vi "Shooter Oper.vi"   [LabVIEW 2016]
uses:
  Robot Global Data.vi
types:
  T1 = typedef "WPI_DriverStationRobotMode2.ctl" = enum16{"Autonomous Disabled", "Autonomous Enabled", "Teleop Disabled", "Teleop Enabled", "Disconnected", "Finish", "Test Disabled", "Test Enabled", "Emergency Stopped"}
  T2 = typedef "WPI_MotorControlDeviceRef.ctl" = cluster{"DeviceStatus":errorcluster, "Type":T3, "PWM":cluster{"PWM Channel":T4, "DeadBand":T5}, "CAN":cluster{"Device Number":u8, "SetOutput VI Ref":variant, "GetOutput VI Ref":variant, "Enable VI Ref":variant, "Disable VI Ref":variant, "Data":variant}, "Invert":bool}
  T3 = typedef "WPI_MotorControlType.ctl" = enum16{"PWM", "CAN"}
  T4 = typedef "FPGA_DIOPWMChannel.ctl" = enum8{"PWM 0", "PWM 1", "PWM 2", "PWM 3", "PWM 4", "PWM 5", "PWM 6", "PWM 7", "PWM 8", "PWM 9", "PWM MXP 0", "PWM MXP 1", "PWM MXP 2", "PWM MXP 3", "PWM MXP 4", "PWM MXP 5", "PWM MXP 6", "PWM MXP 7", "PWM MXP 8", "PWM MXP 9", "Invalid"}
  T5 = typedef "WPI_PWMDeadband.ctl" = cluster{"Name":string, "maxPositivePwm":i32, "minPositivePwm":i32, "centerPwm":i32, "maxNegativePwm":i32, "minNegativePwm":i32, "angularRange":u16}
  T6 = enum16{"Shooter 1 Speed Increase", "Shooter 1 Speed Decrease", "Shooter 2 Speed Increase", "Shooter 2 Speed Decrease", "Nothing Changed", "Set Zero"}
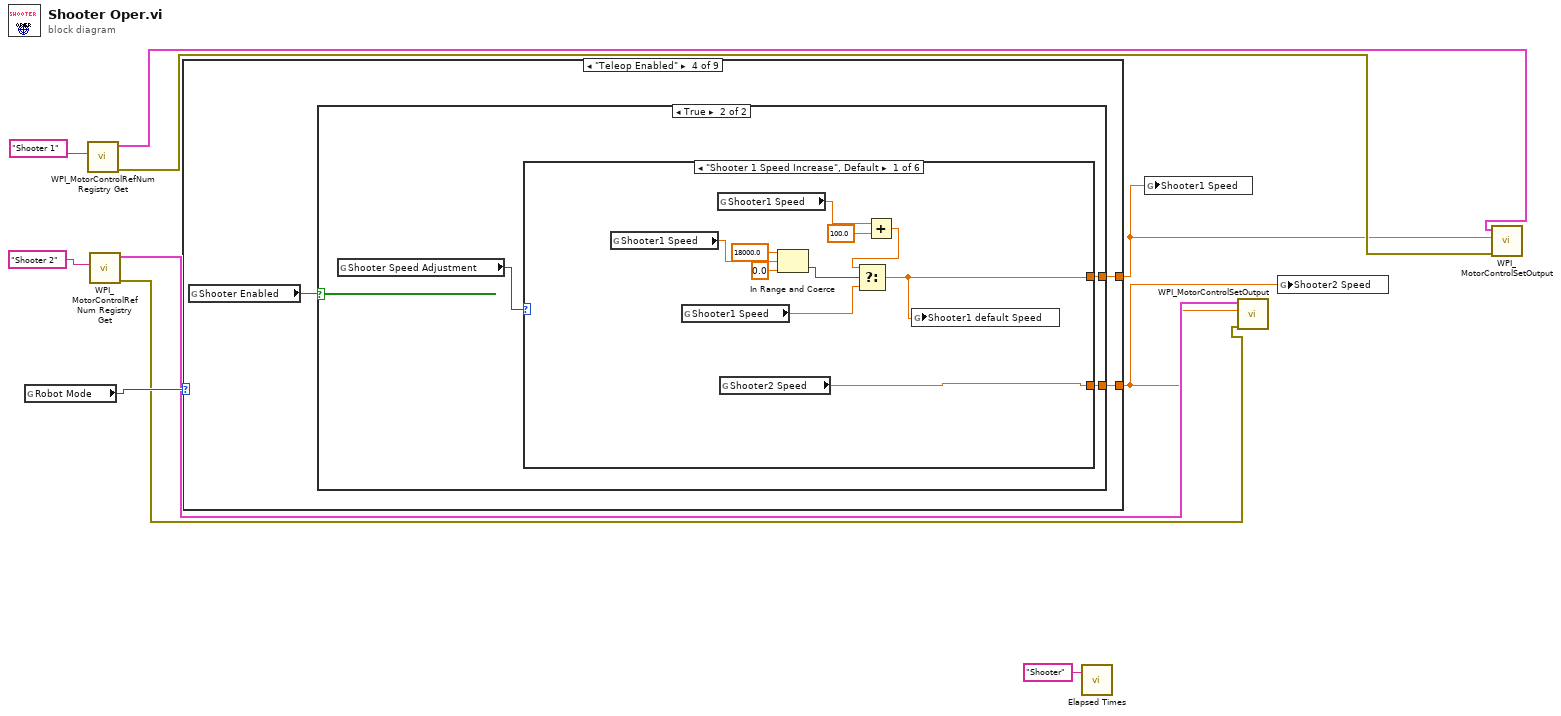
[diagram p0: block diagram]
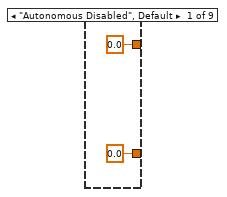
[diagram p2: hidden frame]
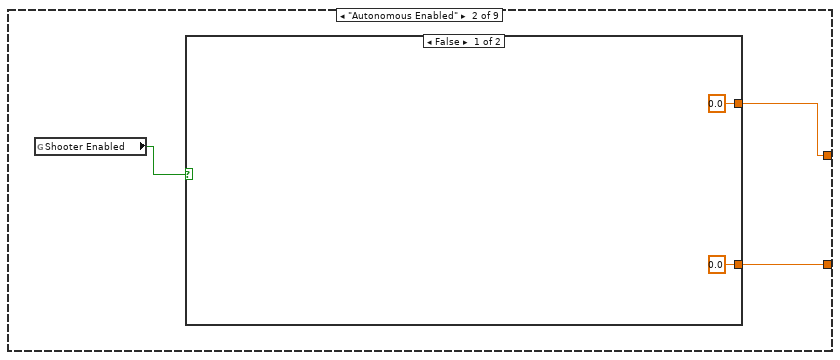
[diagram p3: hidden frame]
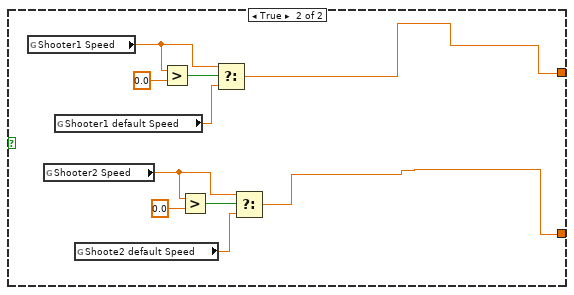
[diagram p4: hidden frame]
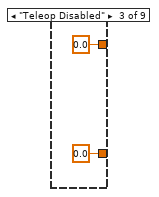
[diagram p5: hidden frame]
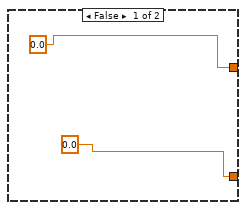
[diagram p6: hidden frame]
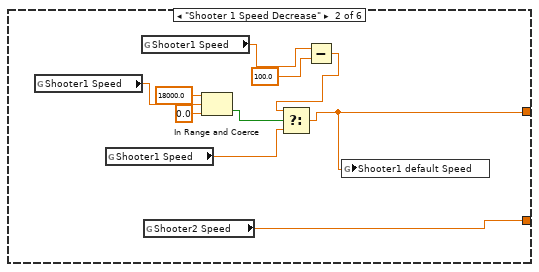
[diagram p7: hidden frame]
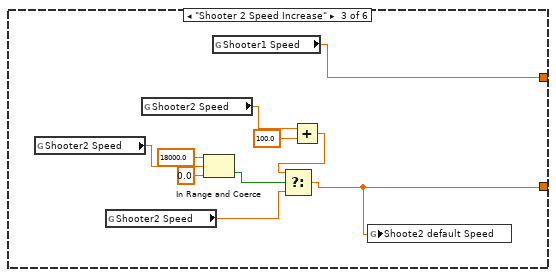
[diagram p8: hidden frame]
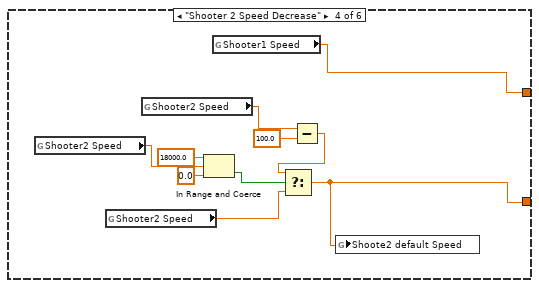
[diagram p9: hidden frame]
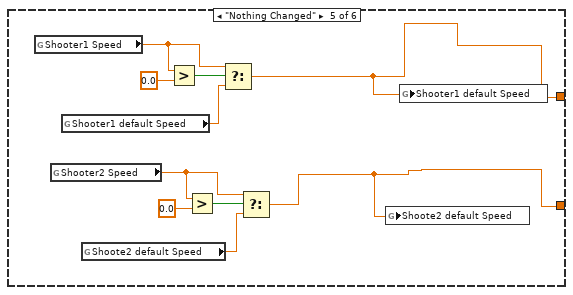
[diagram p10: hidden frame]
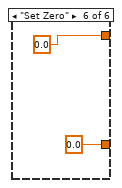
[diagram p11: hidden frame]
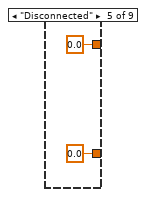
[diagram p12: hidden frame]
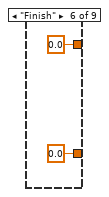
[diagram p13: hidden frame]
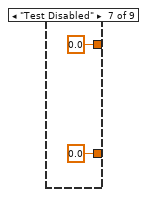
[diagram p14: hidden frame]
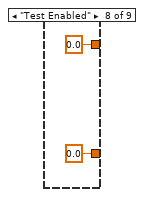
[diagram p15: hidden frame]
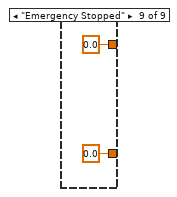
[diagram p16: hidden frame]
diagram:
  n1 = global read "Robot Global Data.vi" "Robot Mode"() -> (w8:T1)
  n2 = call <vilib>:"WPI_MotorControlRefNum Registry Get.vi"("refnum name"="Shooter 1") -> ("error out"=w5:errorcluster, "MotorControlDevRef"=w7:T2)  [unwired: 9 in]
  n3 = call <vilib>:"WPI_MotorControlRefNum Registry Get.vi"("refnum name"="Shooter 2") -> ("error out"=w4:errorcluster, "MotorControlDevRef"=w6:T2)  [unwired: 9 in]
  n4 = case shown="\"Teleop Enabled\"" w8 {
    tunnel: [0.0 ("Shooter1 Speed") w13 0.0 ("Shooter1 Speed") w31 0.0 ("Shooter1 Speed") 0.0 ("Shooter1 Speed") 0.0 ("Shooter1 Speed") 0.0 ("Shooter1 Speed") 0.0 ("Shooter1 Speed")] -> w3
    tunnel: [0.0 ("Shooter2 Speed") w14 0.0 ("Shooter2 Speed") w30 0.0 ("Shooter2 Speed") 0.0 ("Shooter2 Speed") 0.0 ("Shooter2 Speed") 0.0 ("Shooter2 Speed") 0.0 ("Shooter2 Speed")] -> w2
    frame "Autonomous Disabled", Default {
    }
    frame "Autonomous Enabled" {
      n5 = global read "Robot Global Data.vi" "Shooter Enabled"() -> (w15:bool)
      n6 = case shown="False" w15 {
        tunnel: [0.0 ("Shooter2 Speed") w19] -> w14
        tunnel: [0.0 ("Shooter1 Speed") w18] -> w13
        frame False {
        }
        frame True {
          n7 = global read "Robot Global Data.vi" "Shooter1 Speed"() -> (w25:dbl)
          n8 = global read "Robot Global Data.vi" "Shooter2 Speed"() -> (w21:dbl)
          n9 = global read "Robot Global Data.vi" "Shooter1 default Speed"() -> (w24:dbl)
          n10 = global read "Robot Global Data.vi" "Shoote2 default Speed"() -> (w20:dbl)
          n11 = Greater?(x=w25, y=0.0) -> (0:w26:bool)
          n12 = Greater?(x=w21, y=0.0) -> (0:w22:bool)
          n13 = Select(t=w25, s=w26, f=w24) -> (s? t:f=w18:dbl)
          n14 = Select(t=w21, s=w22, f=w20) -> (s? t:f=w19:dbl)
        }
      }
    }
    frame "Teleop Disabled" {
    }
    frame "Teleop Enabled" {
      n15 = global read "Robot Global Data.vi" "Shooter Enabled"() -> (w32:bool)
      n16 = case shown="True" w32 {
        tunnel: [0.0 ("Shooter1 Speed") w36] -> w31
        tunnel: [0.0 ("Shooter2 Speed") w35] -> w30
        frame False {
        }
        frame True {
          n17 = global read "Robot Global Data.vi" "Shooter Speed Adjustment"() -> (w37:T6)
          n18 = case shown="\"Shooter 1 Speed Increase\", Default" w37 {
            tunnel: [w38 w48 w59 w69 w79 0.0 ("Shooter1 Speed")] -> w36
            tunnel: [w39 w49 w58 w68 w78 0.0 ("Shooter2 Speed")] -> w35
            frame "Shooter 1 Speed Increase", Default {
              n19 = global read "Robot Global Data.vi" "Shooter1 Speed"() -> (w47:dbl)
              n20 = global read "Robot Global Data.vi" "Shooter1 Speed"() -> (w43:dbl)
              n21 = global read "Robot Global Data.vi" "Shooter1 Speed"() -> (w42:dbl)
              n22 = global read "Robot Global Data.vi" "Shooter2 Speed"() -> (w39:dbl)
              n23 = In Range and Coerce(upper limit=18000.0, x=w47, lower limit=0.0) -> (In Range?=w44:bool)  [unwired: 1 out]
              n24 = Add(x=w42, y=100.0) -> (x+y=w40:dbl)
              n25 = Select(t=w40, s=w44, f=w43) -> (s? t:f=w38:dbl)
              n26 = global write "Robot Global Data.vi" "Shooter1 default Speed"(w38) -> ()
            }
            frame "Shooter 1 Speed Decrease" {
              n27 = global read "Robot Global Data.vi" "Shooter1 Speed"() -> (w57:dbl)
              n28 = global read "Robot Global Data.vi" "Shooter1 Speed"() -> (w53:dbl)
              n29 = global read "Robot Global Data.vi" "Shooter1 Speed"() -> (w52:dbl)
              n30 = global read "Robot Global Data.vi" "Shooter2 Speed"() -> (w49:dbl)
              n31 = In Range and Coerce(upper limit=18000.0, x=w57, lower limit=0.0) -> (In Range?=w54:bool)  [unwired: 1 out]
              n32 = Subtract(x=w52, y=100.0) -> (x-y=w50:dbl)
              n33 = Select(t=w50, s=w54, f=w53) -> (s? t:f=w48:dbl)
              n34 = global write "Robot Global Data.vi" "Shooter1 default Speed"(w48) -> ()
            }
            frame "Shooter 2 Speed Increase" {
              n35 = global read "Robot Global Data.vi" "Shooter2 Speed"() -> (w67:dbl)
              n36 = global read "Robot Global Data.vi" "Shooter2 Speed"() -> (w63:dbl)
              n37 = global read "Robot Global Data.vi" "Shooter2 Speed"() -> (w62:dbl)
              n38 = In Range and Coerce(upper limit=18000.0, x=w67, lower limit=0.0) -> (In Range?=w64:bool)  [unwired: 1 out]
              n39 = global read "Robot Global Data.vi" "Shooter1 Speed"() -> (w59:dbl)
              n40 = Add(x=w62, y=100.0) -> (x+y=w60:dbl)
              n41 = Select(t=w60, s=w64, f=w63) -> (s? t:f=w58:dbl)
              n42 = global write "Robot Global Data.vi" "Shoote2 default Speed"(w58) -> ()
            }
            frame "Shooter 2 Speed Decrease" {
              n43 = global read "Robot Global Data.vi" "Shooter2 Speed"() -> (w77:dbl)
              n44 = global read "Robot Global Data.vi" "Shooter2 Speed"() -> (w73:dbl)
              n45 = global read "Robot Global Data.vi" "Shooter2 Speed"() -> (w72:dbl)
              n46 = In Range and Coerce(upper limit=18000.0, x=w77, lower limit=0.0) -> (In Range?=w74:bool)  [unwired: 1 out]
              n47 = global read "Robot Global Data.vi" "Shooter1 Speed"() -> (w69:dbl)
              n48 = Subtract(x=w72, y=100.0) -> (x-y=w70:dbl)
              n49 = Select(t=w70, s=w74, f=w73) -> (s? t:f=w68:dbl)
              n50 = global write "Robot Global Data.vi" "Shoote2 default Speed"(w68) -> ()
            }
            frame "Nothing Changed" {
              n51 = global read "Robot Global Data.vi" "Shooter1 Speed"() -> (w85:dbl)
              n52 = global read "Robot Global Data.vi" "Shooter2 Speed"() -> (w81:dbl)
              n53 = global read "Robot Global Data.vi" "Shooter1 default Speed"() -> (w84:dbl)
              n54 = global read "Robot Global Data.vi" "Shoote2 default Speed"() -> (w80:dbl)
              n55 = Greater?(x=w85, y=0.0) -> (0:w86:bool)
              n56 = Greater?(x=w81, y=0.0) -> (0:w82:bool)
              n57 = Select(t=w85, s=w86, f=w84) -> (s? t:f=w79:dbl)
              n58 = Select(t=w81, s=w82, f=w80) -> (s? t:f=w78:dbl)
              n59 = global write "Robot Global Data.vi" "Shoote2 default Speed"(w78) -> ()
              n60 = global write "Robot Global Data.vi" "Shooter1 default Speed"(w79) -> ()
            }
            frame "Set Zero" {
            }
          }
        }
      }
    }
    frame "Disconnected" {
    }
    frame "Finish" {
    }
    frame "Test Disabled" {
    }
    frame "Test Enabled" {
    }
    frame "Emergency Stopped" {
    }
  }
  n61 = call "Elapsed Times.vi"("Call Name"="Shooter") -> ()  [unwired: 2 in, 1 out]
  n62 = global write "Robot Global Data.vi" "Shooter1 Speed"(w3) -> ()
  n63 = call <vilib>:"WPI_MotorControlSetOutput.vi"("error in (no error)"=w4, "Output"=w2, "MotorControlDevRef"=w6) -> ()  [unwired: 6 in, 3 out]
  n64 = global write "Robot Global Data.vi" "Shooter2 Speed"(w2) -> ()
  n65 = call <vilib>:"WPI_MotorControlSetOutput.vi"("error in (no error)"=w5, "Output"=w3, "MotorControlDevRef"=w7) -> ()  [unwired: 6 in, 3 out]
